vi "Pos ctrl window-Buttons disabled state.vi"(8 "error in (no error)":errorcluster, 11 "Disabled":T1(ring)) -> (0 "error out":errorcluster)   [LabVIEW 2020]
uses:
  Globals/Pos ctrl window globals.vi
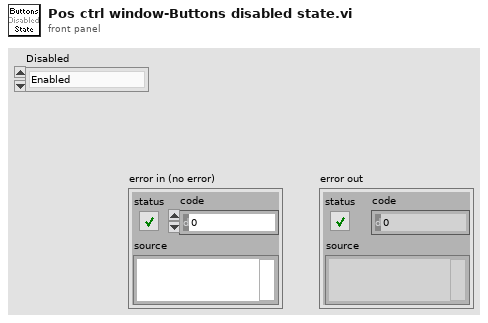
[diagram p1: front panel]
types:
  T1 = enum8{"Enabled", "Disabled", "Disabled and Grayed Out"}
  T2 = typedef "Pos Ctrl window refs cluster.ctl" = cluster{"menu reference":refnum<k9>, "X Coordinate ctrl":refnum<vi>, "Y Coordinate ctrl":refnum<vi>, "Z Coordinate ctrl":refnum<vi>, "Speed setting ctrl":refnum<vi>, "Up":refnum<vi>, "Down":refnum<vi>, "Left":refnum<vi>, "Right":refnum<vi>, "Z move up":refnum<vi>, "Z move down":refnum<vi>, "Down-left":refnum<vi>, "Down-right":refnum<vi>, "Up-left":refnum<vi>, "Up-right":refnum<vi>, "Step = size of image":refnum<vi>, "XY step (um)":refnum<vi>, "Z step (um)":refnum<vi>}
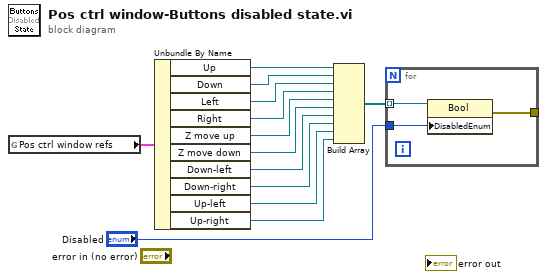
[diagram p0: block diagram]
diagram:
  n1 = global read "Pos ctrl window globals.vi" "Pos ctrl window refs"() -> (w1:T2)
  n2 = Unbundle By Name(w1) -> ("Up"=w2:refnum<vi>, "Down"=w3:refnum<vi>, "Left"=w4:refnum<vi>, "Right"=w5:refnum<vi>, "Z move up"=w6:refnum<vi>, "Z move down"=w7:refnum<vi>, "Down-left"=w8:refnum<vi>, "Down-right"=w9:refnum<vi>, "Up-left"=w10:refnum<vi>, "Up-right"=w11:refnum<vi>)
  n3 = Build Array(w2, w3, w4, w5, w6, w7, w8, w9, w10, w11) -> (w12:refnum<vi>[])
  n4 = for {
    tunnel: w12 -> [w16] mode=indexing
    tunnel: "Disabled" -> [w15]
    tunnel: [w14] -> _
    n5 = property on="Property Node" class="Bool"(reference=w16, "DisabledEnum"=w15) -> (error out=w14:errorcluster)  [unwired: 1 in, 1 out]
  }
